vi "oa_Check Sample Rates of Multi Channel Signals.vi"(2 "error in (no error)":errorcluster, 3 "scaled signals in [EU]":waveform(dbl)[](array[waveform])) -> (0 "error out":errorcluster, 1 "scaled signals out [EU]":waveform(dbl)[](array[waveform]))   [LabVIEW 2017, in "SoundVib_Resampling.lvlib"]
uses:
  <vilib>/addons/Sound and Vibration/Order Analysis/Resample Order Tracking/SoundVib_Resampling.lvlib
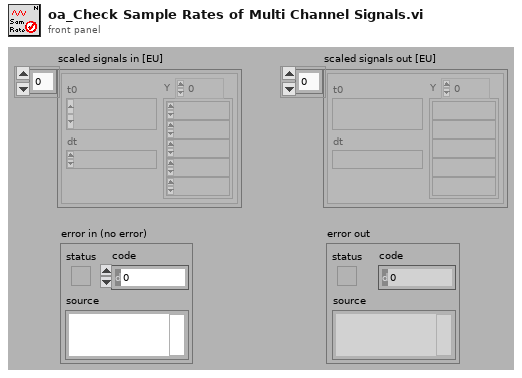
[diagram p1: front panel]
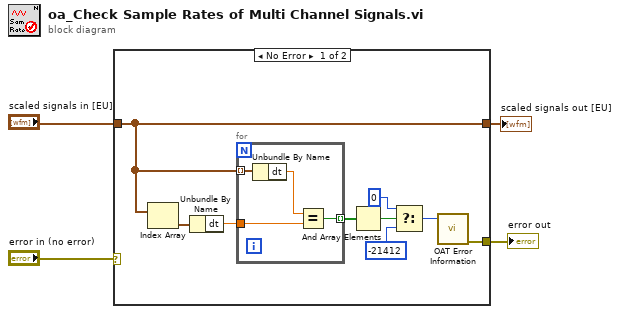
[diagram p0: block diagram]
diagram:
  n1 = case shown="No Error" "error in (no error)" {
    selector: "error in (no error)" -> [_ w19]
    tunnel: [w5 w19] -> w3
    tunnel: "scaled signals in [EU]" -> [w7 w18]
    tunnel: [w7 w18] -> w1
    frame No Error {
      n2 = Index Array(array=w7) -> (element=w13:waveform(dbl))  [unwired: 1 in]
      n3 = Unbundle By Name(w13) -> ("dt"=w12:dbl)
      n4 = for {
        tunnel: w7 -> [w17] mode=indexing
        tunnel: w12 -> [w15]
        tunnel: [w14] -> w11 mode=indexing
        n5 = Unbundle By Name(w17) -> ("dt"=w16:dbl)
        n6 = Equal?(x=w16, y=w15) -> (x = y?=w14:bool)
      }
      n7 = And Array Elements(Boolean array=w11) -> (logical AND=w10:bool)
      n8 = Select(t=0, s=w10, f=-21412) -> (s? t:f=w6:i32)
      n9 = call <vilib>:"OAT Error Information.vi"("error code"=w6) -> ("error out"=w5:errorcluster)  [unwired: 6 in]
    }
    frame Error {
    }
  }
  "error out" <- w3
  "scaled signals out [EU]" <- w1
